vi "Check If Receiver Is Local.vi"(0 "message":T1, 5 "UDP receiver port":u16, 11 "error in":errorcluster) -> (4 "local receiver?":bool, 15 "error out":errorcluster)   [LabVIEW 2009, in "AMC.lvlib"]
doc: "Check if the receiver specified in the message is the same as the local application.\n\nThe receiver is considered local if:\n-\"receiver host\" or \"receiver process\" is empty.\nor\n-\"receiver host\" matches the local IP address and \"UDP reciever port\" matches the local UDP Dispatcher port."
uses:
  AMC.lvlib
  Message.ctl
  <vilib>/NI/Tools/Keyed Array/KeyedArray.ctl
  <vilib>/NI/Tools/Keyed Array/Tools_KeyedArray.lvlib
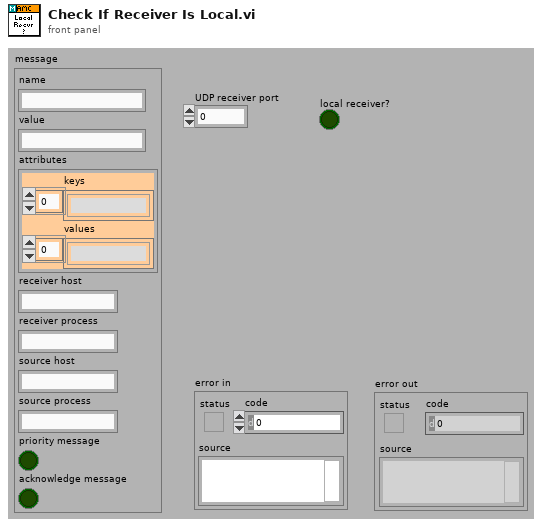
[diagram p1: front panel]
types:
  T1 = typedef "AMC.lvlib/Message.ctl" = cluster{"name":string, "value":string, "attributes":T2, "receiver host":string, "receiver process":string, "source host":string, "source process":string, "priority message":bool, "acknowledge message":bool}
  T2 = typedef "Tools_KeyedArray.lvlib/KeyedArray.ctl" = cluster{"keys":string[], "values":string[]}
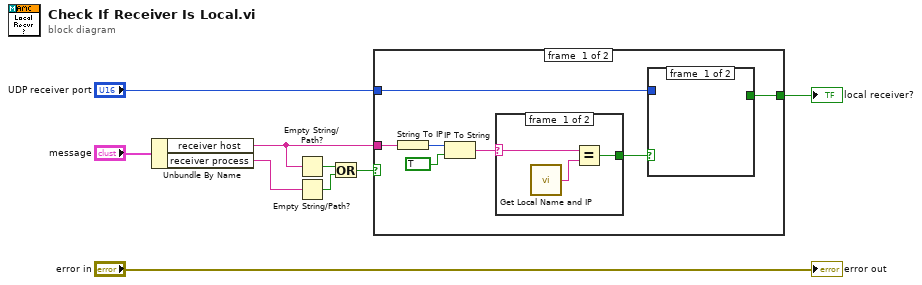
[diagram p0: block diagram]
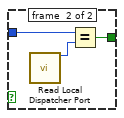
[diagram p2: hidden frame]
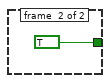
[diagram p3: hidden frame]
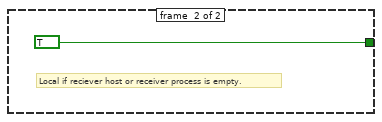
[diagram p4: hidden frame]
diagram:
  n1 = Unbundle By Name("message") -> ("receiver host"=w4:string, "receiver process"=w3:string)
  n2 = Empty String/Path?(string/path=w4) -> (empty?=w6:bool)
  n3 = Empty String/Path?(string/path=w3) -> (empty?=w7:bool)
  n4 = Or(x=w6, y=w7) -> (x .or. y?=w5:bool)
  n5 = case shown="False" w5 {
    tunnel: w4 -> [w16 _]
    tunnel: [w10 TRUE] -> w2
    tunnel: "UDP receiver port" -> [w11 _]
    frame #0 {
      n6 = String To IP(1:w16) -> (0:w14:u32)
      n7 = IP To String(1:TRUE ("dot notation? (F)"), 2:w14) -> (0:w13:string)
      n8 = case shown="\"127.0.0.1\"" w13 {
        selector: w13 -> [w22 _]
        tunnel: [w21 TRUE] -> w12
        frame #0 {
          n9 = call "Get Local Name and IP.vi"() -> ("IP address"=w20:string)  [unwired: 12 in, 3 out]
          n10 = Equal?(x=w22, y=w20) -> (x = y?=w21:bool)
        }
        frame #1 {
        }
      }
      n11 = case shown="True" w12 {
        tunnel: w11 -> [_ w19]
        tunnel: [_ w17] -> w10
        frame #0 {
        }
        frame #1 {
          n12 = call "Read Local Dispatcher Port.vi"() -> ("UDP port"=w18:u16)  [unwired: 14 in, 1 out]
          n13 = Equal?(x=w19, y=w18) -> (x = y?=w17:bool)
        }
      }
    }
    frame #1 {
      # "Local if reciever host or receiver process is empty."
    }
  }
  "local receiver?" <- w2
  "error out" <- "error in"
